vi "CAN Send.vi"() -> ()   [LabVIEW 2014]
uses:
  <vilib>/nican/nican.llb/ncNetAttr.ctl
panel:
  in  "interface":string(combo)="CAN1"
  in  "stop":bool
  in  "Data":u8[](array[numeric])=[1, 2, 3, 4, 5, 6, 7, 8] format="%.0x"
  in  "Set RTR flag?":bool
  in  "Data Length":u32=8 max=8 format="%.0x"
  in  "Arbitration Id":u32=8 format="%.0x"
  in  "Write frame":bool
  in  "Baudrate":u32=125000
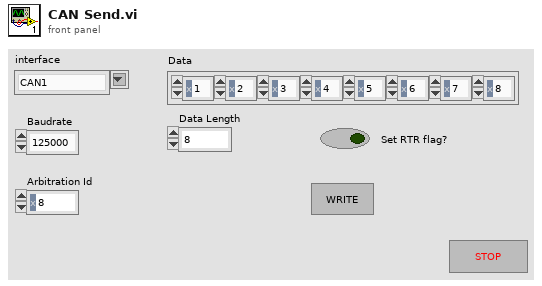
[diagram p1: front panel]
types:
  T1 = typedef "ncNetAttr.ctl" = cluster{"Start On Open":enum32{"FALSE", "TRUE"}, "Baud Rate":u32, "Read Queue Length":u32, "Write Queue Length":u32, "Standard Comparator":u32, "Standard Mask":u32, "Extended Comparator":u32, "Extended Mask":u32}
  T2 = typedef "xobjhandle.ctl" = u32
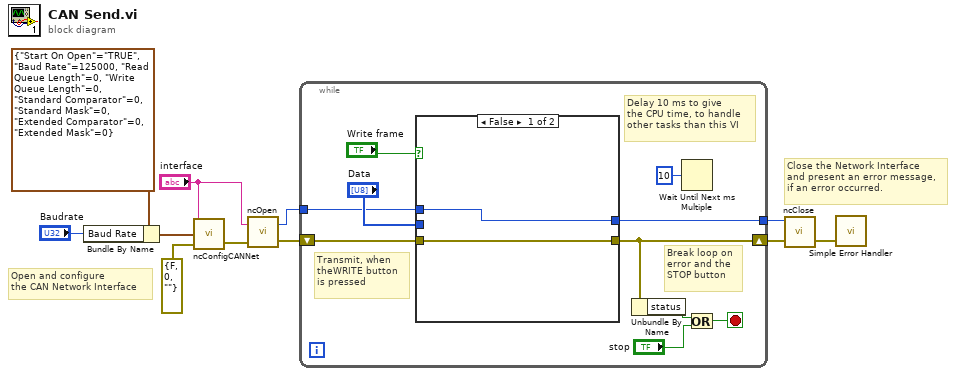
[diagram p0: block diagram]
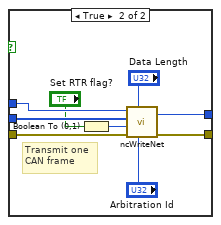
[diagram p2: hidden frame]
diagram:
  # "Open and configure \nthe CAN Network Interface"
  # "Close the Network Interface \nand present an error message, \nif an error occurred."
  n1 = Bundle By Name(cluster=T1 {"Start On Open"=enum."TRUE", "Baud Rate"=125000, "Read Queue Length"=0, "Write Queue Length"=0, "Standard Comparator"=0, "Standard Mask"=0, "Extended Comparator"=0, "Extended Mask"=0} ("CAN Network Interface Config"), "Baud Rate"="Baudrate") -> (w8:T1)
  n2 = call <vilib>:"ncConfigCANNet.vi"("Error in"=errorcluster {"status"=FALSE, "code"=0, "source"=""}, "CAN Network Interface Config"=w8, "ObjName"="interface") -> ("Error out"=w10:errorcluster)  [unwired: 2 in]
  n3 = call <vilib>:"ncOpen.vi"("Error in"=w10, "ObjName"="interface") -> ("Error out"=w4:errorcluster, "ObjHandle out"=w6:T2)
  n4 = while {
    shift-left: w4 -> [w13]
    shift-right: [w12] -> w3
    tunnel: w6 -> [w15]
    tunnel: [w19] -> w5
    stop <- w16 stop-if-true
    # "Transmit, when \ntheWRITE button \nis pressed"
    # "Delay 10 ms to give \nthe CPU time, to handle \nother tasks than this VI"
    # "Break loop on \nerror and the\nSTOP button"
    n5 = case shown="False" "Write frame" {
      tunnel: w15 -> [w22 w31]
      tunnel: w13 -> [w23 w32]
      tunnel: [w23 w30] -> w12
      tunnel: "Data" -> [_ w29]
      tunnel: [w22 w28] -> w19
      frame False {
      }
      frame True {
        # "Transmit one \nCAN frame"
        n6 = Boolean To (0,1)(Boolean="Set RTR flag?") -> (0, 1=w27:i16)
        n7 = call <vilib>:"ncWriteNet.vi"("ArbitrationId"="Arbitration Id", "DataLength"="Data Length", "Error in"=w32, "IsRemote"=w27, "Data"=w29, "ObjHandle in"=w31) -> ("Error out"=w30:errorcluster, "ObjHandle out"=w28:T2)
      }
    }
    n8 = Unbundle By Name(w12) -> ("status"=w18:bool)
    n9 = Wait Until Next ms Multiple(millisecond multiple=u32 10) -> ()  [unwired: 1 out]
    n10 = Or(x=w18, y="stop") -> (x .or. y?=w16:bool)
  }
  n11 = call <vilib>:"ncClose.vi"("Error in"=w3, "ObjHandle in"=w5) -> ("Error out"=w11:errorcluster)  [unwired: 1 in]
  n12 = call <vilib>:"Simple Error Handler.vi"("error in (no error)"=w11) -> ()  [unwired: 4 in, 5 out]
